vi "gentec-SOLO-PE.Tree.vi"   [LabVIEW 2014, in "gentec-SOLO-PE - Driver.lvlib"]
doc: "This is the instrument driver for the gentec SOLO-PE Powermeter. The VI Tree displays all the user-callable VIs of the instrument driver in an organized table."
uses:
  gentec-SOLO-PE - Driver.lvlib
  Driver/Type Defs/gentec-SOLO-PE.Queries with String Answers.ctl
  Driver/Type Defs/gentec-SOLO-PE.Correction Type.ctl
  Driver/Type Defs/gentec-SOLO-PE.Data Sampling Settings.ctl
  Driver/Type Defs/gentec-SOLO-PE.Scale.ctl
  Driver/Type Defs/gentec-SOLO-PE.Enable Statistics.ctl
  Driver/Type Defs/gentec-SOLO-PE.Zero Offset.ctl
panel:
  # "SEE DIAGRAM\nFOR VI TREE."
types:
  T1 = typedef "gentec-SOLO-PE - Driver.lvlib/gentec-SOLO-PE.Zero Offset.ctl" = u32
  T2 = typedef "gentec-SOLO-PE - Driver.lvlib/gentec-SOLO-PE.Enable Statistics.ctl" = u32
  T3 = typedef "gentec-SOLO-PE - Driver.lvlib/gentec-SOLO-PE.Scale.ctl" = u32
  T4 = typedef "gentec-SOLO-PE - Driver.lvlib/gentec-SOLO-PE.Data Sampling Settings.ctl" = cluster{"Sample Rate":u32, "Sample Rate Unit":u32, "Sample Period":u32, "Sample Period Unit":u32, "Total Duration":u32, "Total Duration Unit":u32, "Time Stamp":u32}
  T5 = typedef "gentec-SOLO-PE - Driver.lvlib/gentec-SOLO-PE.Correction Type.ctl" = u16
  T6 = typedef "gentec-SOLO-PE - Driver.lvlib/gentec-SOLO-PE.Queries with String Answers.ctl" = string
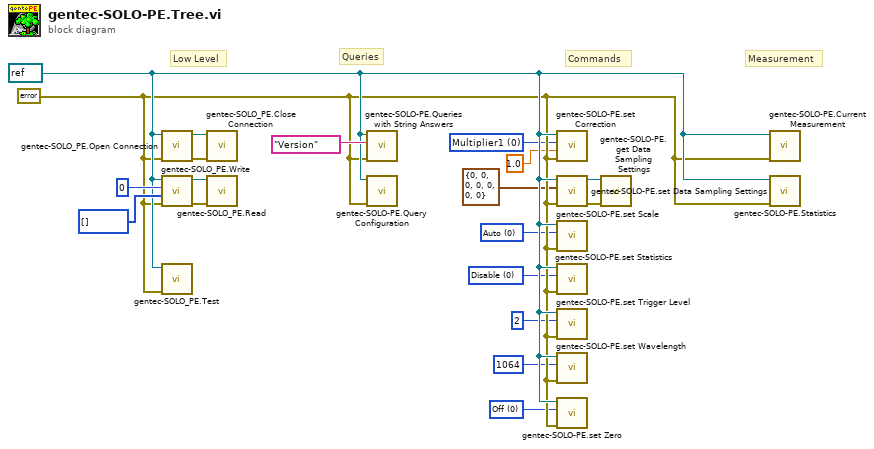
[diagram p0: block diagram]
diagram:
  w1 = T1 0 items=["Off", "On", "Undo"] ("Zero Offset Operation")
  w4 = T2 0 items=["Disable", "Enable", "Reset"] ("Enable Statistics")
  w5 = T3 0 items=["Auto", "1 pJ", "3 pJ", "10 pJ", "30 pJ", "100 pJ", "300 pJ", "1 nJ", "3 nJ", "10 nJ", "30 nJ", "100 nJ", "300 nJ", "1 uJ", "3 uJ", "10 uJ", "30 uJ", "100 uJ", "300 uJ", "1 mJ", "3 mJ", "10 mJ", "30 mJ", "100 mJ", "300 mJ", "1 J", "3 J", "10 J", "30 J", "100 J", "300 J", "1 kJ", "3 kJ", "10 kJ", "30 kJ", "100 kJ", "300 kJ", "1 MJ", "3 MJ", "10 MJ", "30 MJ", "100 MJ", "300 MJ"] ("Scale")
  w8 = T5 0 items=["Multiplier1", "Offset 1", "Multiplier 2", "Offset 2"] ("Correction Type")
  w9 = errorcluster {"status"=FALSE, "code"=0, "source"=""} ("error in")
  w12 = refnum<visa-resource-name> refnum ("VISA resource In")
  # "Measurement"
  # "Commands"
  # "Queries"
  # "Low Level"
  n1 = call "gentec-SOLO_PE.Open Connection.vi"("error in"=w9, "VISA resource name in"=w12) -> ("error out"=w16:errorcluster, "VISA resource name out"=w17:refnum<visa-resource-name>)  [unwired: 3 in, 1 out]
  n2 = call "gentec-SOLO_PE.Write.vi"("error in (no error)"=w9, "Parameters (Empty)"=u32[] [], "Command Handle"=u16 0, "VISA Refnum in"=w12) -> ("error out"=w15:errorcluster, "VISA Refnum out"=w18:refnum<visa-resource-name>)  [unwired: 6 in]
  n3 = call "gentec-SOLO_PE.Test.vi"("error in (no error)"=w9, "VISA Refnum in"=w12) -> ()  [unwired: 5 in, 5 out]
  n4 = call "gentec-SOLO_PE.Close Connection.vi"("error in"=w16, "VISA resource name in"=w17) -> ()  [unwired: 5 in, 1 out]
  n5 = call "gentec-SOLO_PE.Read.vi"("error in (no error)"=w15, "VISA Refnum in"=w18) -> ()  [unwired: 5 in, 5 out]
  n6 = call "gentec-SOLO-PE.Queries with String Answers.vi"("error in (no error)"=w9, "Queries with String Answers"=T6 "Version", "VISA Refnum in"=w12) -> ()  [unwired: 4 in, 5 out]
  n7 = call "gentec-SOLO-PE.Query Configuration.vi"("error in (no error)"=w9, "VISA Refnum in"=w12) -> ()  [unwired: 5 in, 5 out]
  n8 = call "gentec-SOLO-PE.set Correction.vi"("error in (no error)"=w9, "Correction Value"=1.0, "Correction Type"=w8, "VISA Refnum in"=w12) -> ()  [unwired: 3 in, 5 out]
  n9 = call "gentec-SOLO-PE.set Data Sampling Settings.vi"("error in (no error)"=w9, "Data Samling Settings"=T4 {"Sample Rate"=0, "Sample Rate Unit"=0, "Sample Period"=0, "Sample Period Unit"=0, "Total Duration"=0, "Total Duration Unit"=0, "Time Stamp"=0}, "VISA Refnum in"=w12) -> ("error out"=w10:errorcluster, "VISA Refnum out"=w11:refnum<visa-resource-name>)  [unwired: 4 in, 3 out]
  n10 = call "gentec-SOLO-PE.set Scale.vi"("error in (no error)"=w9, "Scale"=w5, "VISA Refnum in"=w12) -> ()  [unwired: 4 in, 5 out]
  n11 = call "gentec-SOLO-PE.set Statistics.vi"("error in (no error)"=w9, "Enable Statistics"=w4, "VISA Refnum in"=w12) -> ()  [unwired: 4 in, 5 out]
  n12 = call "gentec-SOLO-PE.set Trigger Level.vi"("error in (no error)"=w9, "Trigger Level (2%)"=u32 2, "VISA Refnum in"=w12) -> ()  [unwired: 4 in, 5 out]
  n13 = call "gentec-SOLO-PE.set Wavelength.vi"("error in (no error)"=w9, "Wavelength [nm]"=u32 1064, "VISA Refnum in"=w12) -> ()  [unwired: 4 in, 5 out]
  n14 = call "gentec-SOLO-PE.set Zero.vi"("error in (no error)"=w9, "Zero Offset Operation"=w1, "VISA Refnum in"=w12) -> ()  [unwired: 4 in, 5 out]
  n15 = call "gentec-SOLO-PE.get Data Sampling Settings.vi"("error in (no error)"=w10, "VISA Refnum in"=w11) -> ()  [unwired: 5 in, 5 out]
  n16 = call "gentec-SOLO-PE.Current Measurement.vi"("error in (no error)"=w9, "VISA Refnum in"=w12) -> ()  [unwired: 4 in, 6 out]
  n17 = call "gentec-SOLO-PE.Statistics.vi"("error in (no error)"=w9, "VISA Refnum in"=w12) -> ()  [unwired: 5 in, 5 out]
